vi "Program Start.vi"() -> (0 "error out":errorcluster, 3 "user events":refnum<queue>, 4 "objects":T1, 5 "Event Registration Refnum out":refnum<event-registration>, 6 "user interface":refnum<queue>, 7 "user event":refnum<user-event>)   [LabVIEW 2011]
uses:
  Controls/User Interface Control.ctl
  Controls/User Interface Action.ctl
  Controls/User Event Control.ctl
  Controls/User Event Action.ctl
  Controls/Class Objects.ctl
  Modules/File/Configuration/Configuration.lvclass
  Modules/Hardware/Power Supply/Power Supply.lvclass
  Modules/Hardware/Mass Flow Controller/Mass Flow Controller.lvclass
  Modules/Hardware/Valve Controller/Valve Controller.lvclass
  Modules/Hardware/Multimeter/Multimeter.lvclass
  Modules/Hardware/Vapour Generator/Vapour Generator.lvclass
  Modules/File/TDMS/TDMS.lvclass
  Modules/Hardware/PID/PID.lvclass
  Error Handling/Error Module Action.ctl
  Functional Global Data/User Interface Global.ctl
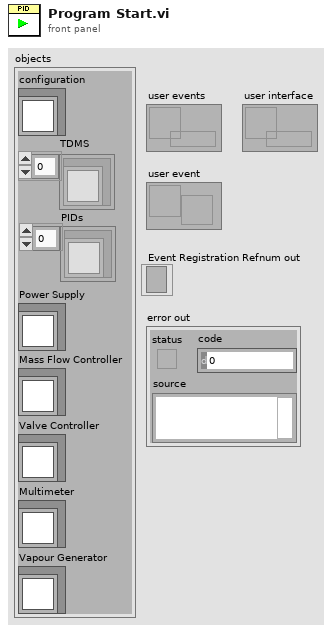
[diagram p1: front panel]
types:
  T1 = typedef "Class Objects.ctl" = cluster{"configuration":refnum<class "Configuration.lvclass">, "TDMS":refnum<class "TDMS.lvclass">[], "Power Supply":refnum<class "Power Supply.lvclass">, "Mass Flow Controller":refnum<class "Mass Flow Controller.lvclass">, "Valve Controller":refnum<class "Valve Controller.lvclass">, "Multimeter":refnum<class "Multimeter.lvclass">, "Vapour Generator":refnum<class "Vapour Generator.lvclass">, "PIDs":refnum<class "PID.lvclass">[]}
  T2 = typedef "User Interface Global.ctl" = enum16{"Initialize", "Update UI", "Stop"}
  T3 = typedef "User Interface Control.ctl" = cluster{"action":T4, "data1":variant, "data2":variant}
  T4 = typedef "User Interface Action.ctl" = enum16{"Initialize", "Data Acquisition Disable", "Data View Disable", "Sample Set", "Sample Set 2D Data", "Sample Set x0 & dx", "Sample Add", "Sample Set Cursor", "Sample Set Offset & Multiplier", "Sample Set Axis Labels", "Sample Parameters Disabled", "Sample Parameters Update", "Run Update", "Run Set Offset & Multiplier", "Run Set Axis Labels", "Run Set Cursor", "Run Set Disabled", "Run Parameters Update", "Run Parameters Disabled", "Run Number Set", "Run Number Set Range", "Run Number Set Disabled", "Sample Number Set", "Sample Number Set Range", "Notes Set Value", "Update Plot", "Set Plot Parameters", "Update Concentration Plot", "Time Set", "Clear DAQ Display", "Clear Analysis Display", "Status Bar Set", "Progress Bar Set", "Display Mode Set", "Experiment Type Set", "Analysis Plot Average Set", "Stop"}
  T5 = typedef "User Event Control.ctl" = cluster{"action":T6, "data":variant}
  T6 = typedef "User Event Action.ctl" = enum16{"Program Initialization", "Device Connections", "Device Settings", "Options", "DAQ Init", "PID Sample Test", "PID with PS Challenge", "PID with MFC Challenge", "Multimeter Sample Test", "Multimeter with MFC Challenge", "DAQ Stop", "Open Data File", "View Data File", "Change Display Mode", "Load INL PID Run Data", "Load Baseline-Mocon PID Data", "Load Multimeter Data", "Set Channel Sample", "Key Down", "Add Spectrum to Plot", "Add History to Plot", "Export History to Excel", "Clear Plots", "Save Plot", "Save Spectral Variable", "History Cursor Release", "Analysis Plot Cursor Release", "Program Deinitialization"}
  T7 = typedef "Error Module Action.ctl" = enum16{"Initialize", "Handle Errors", "Report Errors"}
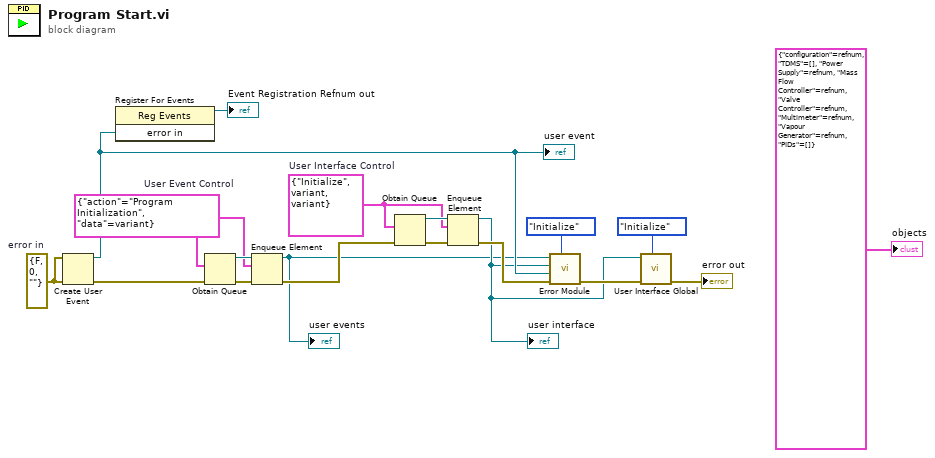
[diagram p0: block diagram]
diagram:
  w10 = T3 {"action"=enum."Initialize", "data1"=variant, "data2"=variant}  # User Interface Control
  w11 = T5 {"action"=enum."Program Initialization", "data"=variant}  # User Event Control
  w19 = errorcluster {"status"=FALSE, "code"=0, "source"=""}  # error in
  n1 = Create User Event(user event datatype=w19, error in=w19) -> (user event=w8:refnum<user-event>, error out=w18:errorcluster)
  "user event" <- w8
  n2 = register-events(w8) -> (reference out=→"Event Registration Refnum out":refnum<event-registration>)  [unwired: 2 in, 1 out]
  n3 = Obtain Queue(element data type=w11, error in (no error)=w18) -> (queue out=w15:refnum<queue>, error out=w14:errorcluster)  [unwired: 3 in, 1 out]
  n4 = Enqueue Element(queue=w15, element=w11, error in (no error)=w14) -> (queue out=w1:refnum<queue>, error out=w12:errorcluster)  [unwired: 1 in, 1 out]
  "user events" <- w1
  n5 = Obtain Queue(element data type=w10, error in (no error)=w12) -> (queue out=w17:refnum<queue>, error out=w16:errorcluster)  [unwired: 3 in, 1 out]
  n6 = Enqueue Element(queue=w17, element=w10, error in (no error)=w16) -> (queue out=w2:refnum<queue>, error out=w7:errorcluster)  [unwired: 1 in, 1 out]
  "user interface" <- w2
  n7 = call "Error Module.vi"("Command (Handle Errors"=Error_Module_Action."Initialize", "error in"=w7, "dynamic event queue reference"=w8, "User Interface Queue Reference"=w2, "User Event Queue Refence"=w1) -> ("error out"=w6:errorcluster)  [unwired: 5 in, 1 out]
  n8 = call "User Interface Global.vi"("command (Update UI)"=User_Interface_Global."Initialize" ("command"), "error in"=w6, "user interface queue reference"=w2) -> ("error out"=→"error out":errorcluster)  [unwired: 8 in]
  "objects" <- T1 {"configuration"=refnum, "TDMS"=[], "Power Supply"=refnum, "Mass Flow Controller"=refnum, "Valve Controller"=refnum, "Multimeter"=refnum, "Vapour Generator"=refnum, "PIDs"=[]} ("objects")
